vi "File_creation.vi"(8 "error in (no error)":errorcluster, 10 "Array of Waveforms":waveform(dbl)[](array[waveform]), 11 "Log File in":refnum<k34>) -> (0 "error out":errorcluster, 3 "Log File out":refnum<k34>)   [LabVIEW 2017]
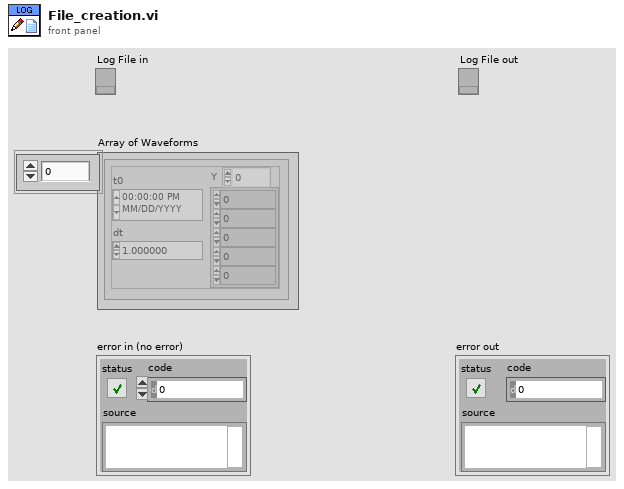
[diagram p1: front panel]
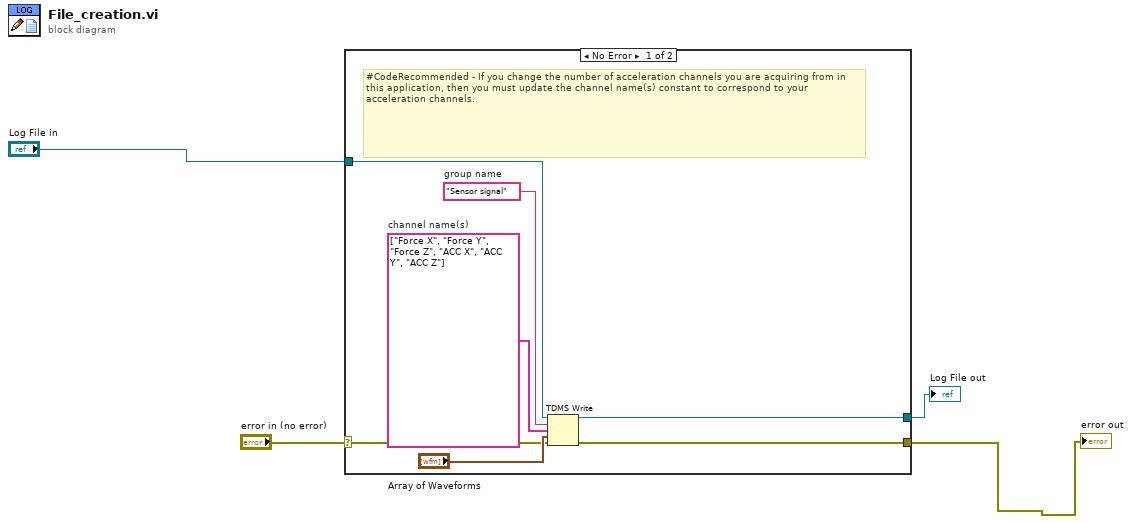
[diagram p0: block diagram]
diagram:
  n1 = case shown="No Error" "error in (no error)" {
    selector: "error in (no error)" -> [w6 w12]
    tunnel: "Log File in" -> [w8 w13]
    tunnel: [w7 w13] -> w3
    tunnel: [w5 w12] -> w1
    frame No Error {
      w9 = string[] ["Force X", "Force Y", "Force Z", "ACC X", "ACC Y", "ACC Z"]  # channel name(s)
      w11 = "Sensor signal"  # group name
      # "#CodeRecommended - If you change the number of acceleration channels you are acquiring from in this application, then you must update the channel name(s) constant to correspond to your acceleration channels."
      n2 = TDMS Write(0:w8, 5:w11, 7:w9, 9:"Array of Waveforms", 11:w6) -> (4:w7:refnum<k34>, 15:w5:errorcluster)  [unwired: 1 in, 2 out]
    }
    frame Error {
    }
  }
  "Log File out" <- w3
  "error out" <- w1
